vi "average_images.vi"(8 "error in (no error)":errorcluster, 10 "Hamamatsu_C9100-13 (in)":refnum<class "Hamamatsu_C9100-13.lvclass">) -> (0 "error out":errorcluster, 2 "Hamamatsu_C9100-13 out":refnum<class "Hamamatsu_C9100-13.lvclass">, 3 "Average of Images":T1(plugin-control))   [LabVIEW 2013]
uses:
  Camera/Hamamatsu_C9100-13/Hamamatsu_C9100-13.lvclass
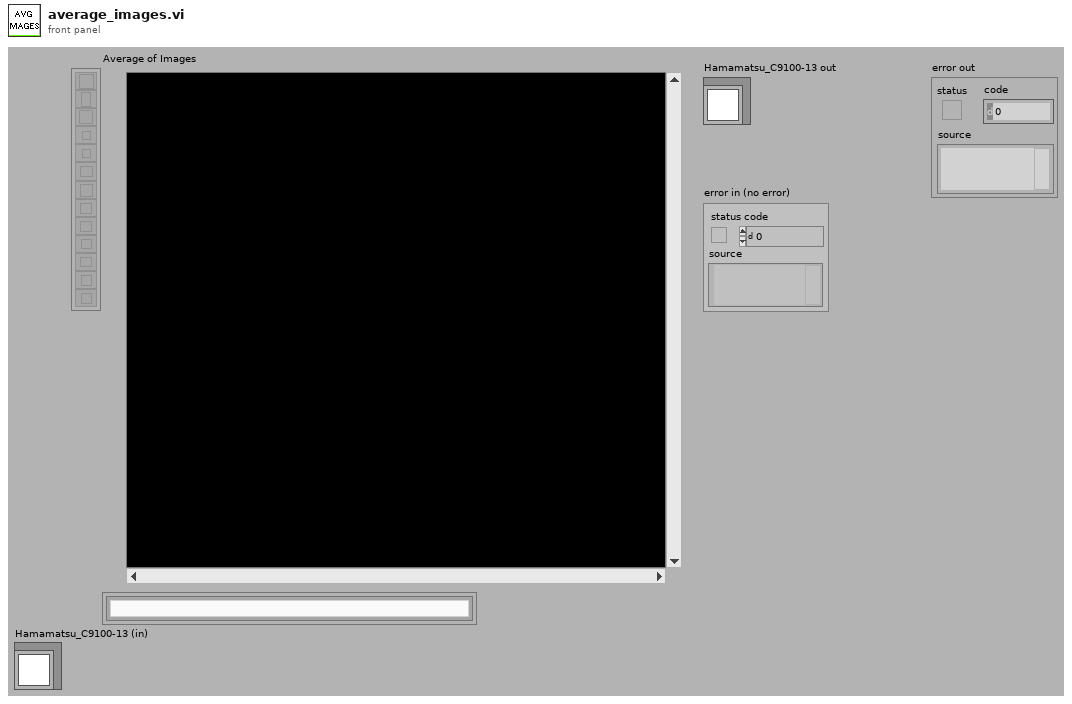
[diagram p1: front panel]
types:
  T1 = typedef "IMAQ Image.ctl" = refnum<image>
  T2 = typedef "Image Type" = u32
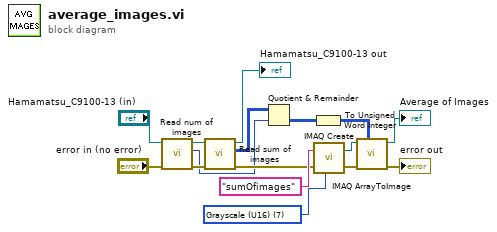
[diagram p0: block diagram]
diagram:
  w12 = T2 7 items=["Grayscale (U8)", "Grayscale (I16)", "Grayscale (SGL)", "Complex (CSG)", "RGB (U32)", "HSL (U32)", "RGB (U64)", "Grayscale (U16)"] ("Image Type")
  n1 = call-dynamic "Read num of images.vi"("error in (no error)"="error in (no error)", "Camera in"="Hamamatsu_C9100-13 (in)") -> ("error out"=w3:errorcluster, "# of images"=w1:u32, "Camera out"=w5:refnum<class "Hamamatsu_C9100-13.lvclass">)  [unwired: 7 in]
  n2 = call-dynamic "Read sum of images.vi"("error in (no error)"=w3, "Camera in"=w5) -> ("error out"=w7:errorcluster, "sum of images"=w2:u32[][], "Camera out"=→"Hamamatsu_C9100-13 out":refnum<class "Hamamatsu_C9100-13.lvclass">)  [unwired: 7 in]
  n3 = Quotient & Remainder(x=w2, y=w1) -> (floor(x/y)=w10:u32[][])  [unwired: 1 out]
  n4 = To Unsigned Word Integer(number=w10) -> (unsigned 16bit integer=w13:u16[][])
  n5 = call "IMAQ Create"("Image Name"="sumOfimages", "Image Type"=w12, "error in (no error)"=w7) -> ("New Image"=w15:T1, "error out"=w14:errorcluster)  [unwired: 2 in]
  n6 = call "IMAQ ArrayToImage"("Image Pixels (U16)"=w13, "error in (no error)"=w14, "Image"=w15) -> ("error out"=→"error out":errorcluster, "Image Out"=→"Average of Images":T1)  [unwired: 7 in]
